vi "HP3458A Open.vi"(8 "error in (no error)":errorcluster, 11 "session in":T1={"VISA"="", "ac method"=0, " resolution"=enum."6.5", "function"=0, "frequency source"=3, "auto range"=1, "manual range"=1.0} {"manual range" format="%_3g"; "auto range" items=["OFF", "ON", "ONCE"]; "frequency source" items=["AC + DC Current", "AC + DC Voltage", "AC Current", "AC Voltage"]; "function" items=["DC Voltage", "AC Voltage", "AC + DC Voltage", "DC Current", "AC Current", "AC + DC Current", "2-Wire Resistance", "4-Wire Resistance", "Frequency", "Period", "Direct Sampling DC", "Direct Sampling AC", "Sub-Sampling DC", "Sub-Sampling AC"]; "ac method" items=["Analog", "Random", "Synchronous"]}) -> (0 "error out":errorcluster, 2 "idn string":string, 3 "session out":T1={"VISA"="", "ac method"=0, " resolution"=enum."6.5", "function"=0, "frequency source"=3, "auto range"=1, "manual range"=1.0} {"manual range" format="%_3g"; "auto range" items=["OFF", "ON", "ONCE"]; "frequency source" items=["AC + DC Current", "AC + DC Voltage", "AC Current", "AC Voltage"]; "function" items=["DC Voltage", "AC Voltage", "AC + DC Voltage", "DC Current", "AC Current", "AC + DC Current", "2-Wire Resistance", "4-Wire Resistance", "Frequency", "Period", "Direct Sampling DC", "Direct Sampling AC", "Sub-Sampling DC", "Sub-Sampling AC"]; "ac method" items=["Analog", "Random", "Synchronous"]})   [LabVIEW 2020]
uses:
  HP3458A Session.ctl
  Agilent 3458.lvlib
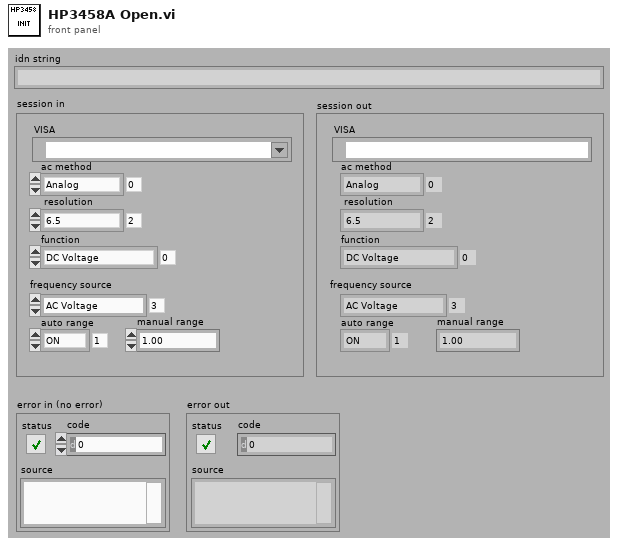
[diagram p1: front panel]
types:
  T1 = typedef "HP3458A Session.ctl" = cluster{"VISA":refnum<visa-resource-name>, "ac method":u16, " resolution":enum16{"4.5", "5.5", "6.5", "7.5", "8.5"}, "function":u16, "frequency source":u16, "auto range":u16, "manual range":dbl}
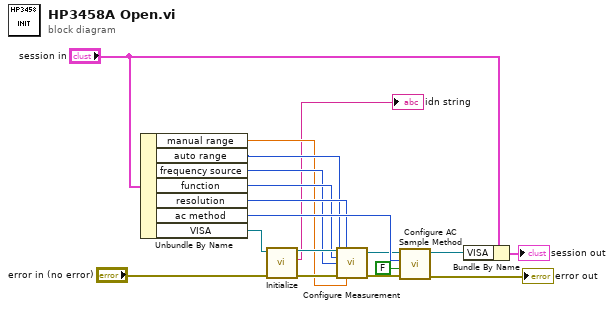
[diagram p0: block diagram]
diagram:
  n1 = Unbundle By Name("session in") -> ("manual range"=w7:dbl, "auto range"=w8:u16, "frequency source"=w9:u16, "function"=w10:u16, "resolution"=w11:enum16{"4.5", "5.5", "6.5", "7.5", "8.5"}, "ac method"=w16:u16, "VISA"=w17:refnum<visa-resource-name>)
  n2 = call "Initialize.vi"("error in (no error)"="error in (no error)", "VISA resource name"=w17) -> ("error out"=w15:errorcluster, "idn string"=→"idn string":string, "VISA resource name out"=w12:refnum<visa-resource-name>)  [unwired: 7 in]
  n3 = call "Configure Measurement.vi"("VISA resource name"=w12, "Manual Resolution (2: 6.5 digits)"=w11, "Function (0: DC Voltage)"=w10, "Frequency Source (3: AC Voltage)"=w9, "Auto Range (1:ON)"=w8, "error in (no error)"=w15, "Manual Range (1.00)"=w7) -> ("VISA resource name out"=w13:refnum<visa-resource-name>, "error out"=w14:errorcluster)  [unwired: 7 in]
  n4 = call "Configure AC Sample Method.vi"("error in (no error)"=w14, "Enable Ratio Measurement(Enable)"=FALSE, "AC Sample Method (0: Analog)"=w16, "VISA resource name"=w13) -> ("error out"=→"error out":errorcluster, "VISA resource name out"=w4:refnum<visa-resource-name>)  [unwired: 6 in]
  n5 = Bundle By Name(cluster="session in", "VISA"=w4) -> (→"session out":T1)
